vi "Atualiza_prioridades_client.vi"(8 "error in":errorcluster, 10 "padrao_prioridade_TAGs_entrada":T1, 11 "refnum in":T2) -> (0 "error out":errorcluster, 2 "padrao_prioridade_TAGs_saida":T1, 3 "refnum out":T2)   [LabVIEW 2019]
uses:
  <vilib>/Utility/config.llb/Config Data RefNum.ctl
  padrao_TAGS_prioridades_client.ctl
  <vilib>/Utility/config.llb/Read Key (Boolean).vi
  <vilib>/Utility/config.llb/NI_LVConfig.lvlib
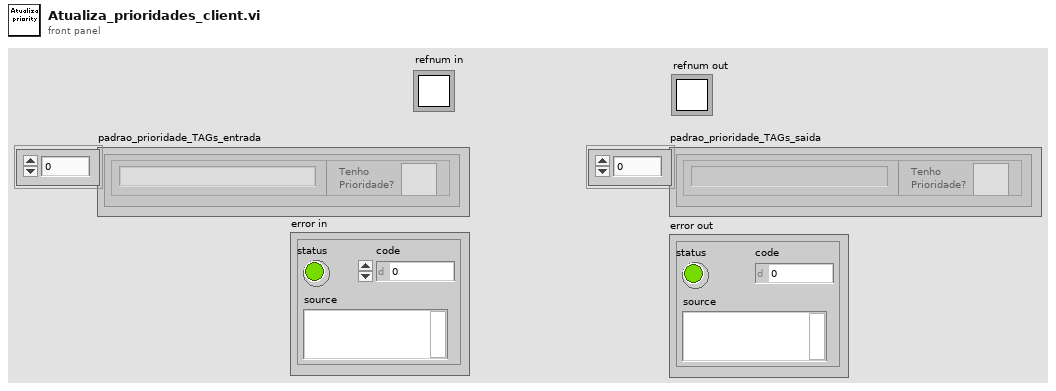
[diagram p1: front panel]
types:
  T1 = typedef "padrao_TAGS_prioridades_client.ctl" = cluster{"TAG":string, "Tenho\nPrioridade?":bool}[]
  T2 = typedef "NI_LVConfig.lvlib/Config Data RefNum.ctl" = refnum<k1>
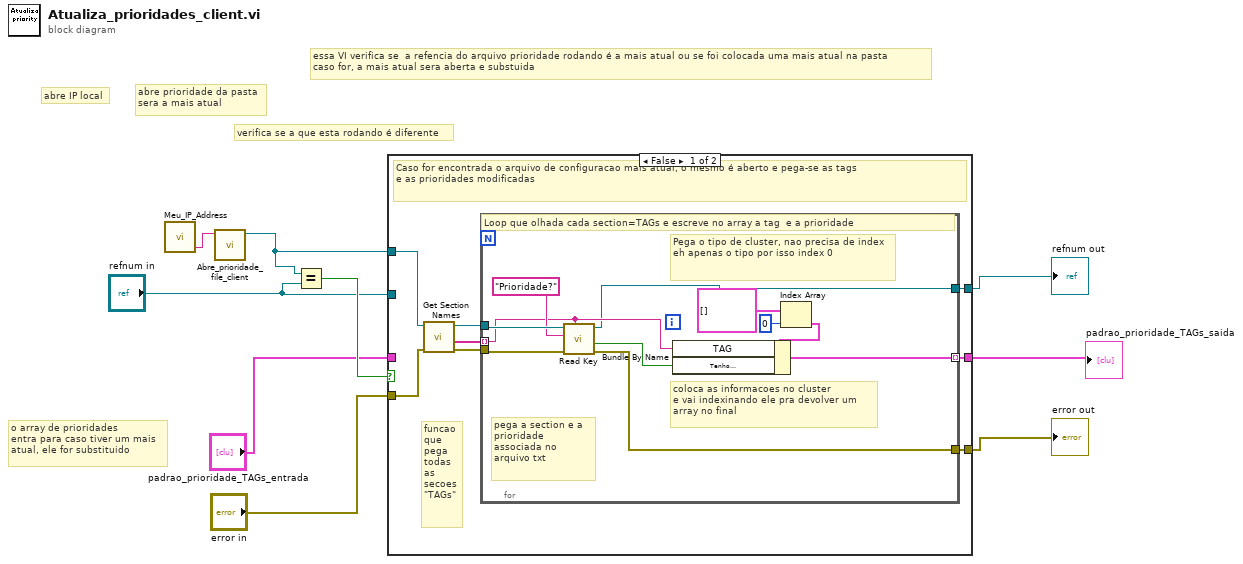
[diagram p0: block diagram]
diagram:
  # "o array de prioridades \nentra para caso tiver um mais\natual, ele for substituido"
  # "verifica se a que esta rodando é diferente"
  # "abre prioridade da pasta\nsera a mais atual"
  # "abre IP local"
  # "essa VI verifica se  a refencia do arquivo prioridade rodando é a mais atual ou se foi colocada uma mais atual na pasta\ncaso for, a mais atual sera aberta e substuida"
  n1 = call "Meu_IP_Address.vi"() -> ("Meu IP"=w6:string)  [unwired: 4 in, 1 out]
  n2 = call "Abre_prioridade_file_client.vi"("Meu_Ip"=w6) -> ("refnum"=w1:T2)  [unwired: 9 in, 1 out]
  n3 = Equal?(x=w1, y="refnum in") -> (x = y?=w5:bool)
  n4 = case shown="False" w5 {
    tunnel: [w17 w30] -> w9
    tunnel: [w16 w31] -> w8
    tunnel: [w15 w29] -> w7
    tunnel: "error in" -> [w14 w31]
    tunnel: "refnum in" -> [_ w30]
    tunnel: "padrao_prioridade_TAGs_entrada" -> [_ w29]
    tunnel: w1 -> [w10 _]
    frame False {
      # "funcao\nque \npega\ntodas \nas\nsecoes\n\"TAGs\""
      # "Caso for encontrada o arquivo de configuracao mais atual, o mesmo é aberto e pega-se as tags\ne as prioridades modificadas"
      n5 = call <vilib>:"Get Section Names.vi"("error in (no error)"=w14, "refnum"=w10) -> ("error out"=w13:errorcluster, "section names"=w12:string[], "refnum out"=w11:T2)  [unwired: 7 in]
      n6 = for {
        tunnel: w12 -> [w26] mode=indexing
        tunnel: w11 -> [w28]
        tunnel: w13 -> [w23]
        tunnel: [w24] -> w15 mode=indexing
        tunnel: [w22] -> w17
        tunnel: [w21] -> w16
        # "coloca as informacoes no cluster \ne vai indexinando ele pra devolver um \narray no final"
        # "Pega o tipo de cluster, nao precisa de index eh apenas o tipo por isso index 0"
        # "pega a section e a prioridade associada no arquivo txt"
        # "Loop que olhada cada section=TAGs e escreve no array a tag  e a prioridade"
        n7 = call-poly <vilib>:"Read Key.vi"("section"=w26, "error in (no error)"=w23, "key"="Prioridade?", "refnum"=w28) -> ("error out"=w21:errorcluster, "value"=w25:bool, "refnum out"=w22:T2)  [unwired: 4 in, 1 out]
        n8 = Index Array(array=T1 [] ("padrao_prioridade_TAGs"), index=0) -> (element=w18:cluster{"TAG":string, "Tenho\nPrioridade?":bool})
        n9 = Bundle By Name(cluster=w18, "TAG"=w26, "Tenho\nPrioridade?"=w25) -> (w24:cluster{"TAG":string, "Tenho\nPrioridade?":bool})
      }
    }
    frame True {
      # "Nao tem moficacao, o fluxo segue normalmente"
    }
  }
  "padrao_prioridade_TAGs_saida" <- w7
  "refnum out" <- w9
  "error out" <- w8
